vi "Pneumatics.vi"(7 "Solenoid Module":T2={"Unassigned"=enum."Solenoid 1", "Unassigned"=enum."Solenoid 2", "Arm In"=enum."Solenoid 3", "Arm Out"=enum."Solenoid 4", "MiniBot In"=enum."Solenoid 5", "MiniBot Out"=enum."Solenoid 6", "Unassigned"=enum."Solenoid 7", "Unassigned"=enum."Solenoid 8", "Switch and Relay Module"=enum."Solenoid Module 1"}, 8 "Mode":enum16{"Init", "Run", "End"}(ring), 10 "Inputs":T1) -> ()   [LabVIEW 2013]
doc: "This VI sets the pneumatics directly."
uses:
  Type Defs/Solenoid Module.ctl
  <vilib>/Rock Robotics/WPI/Solenoid/WPI_SolenoidChannel.ctl
  <vilib>/Rock Robotics/SystemInterfaces/Typedef/FPGA_TypedefSolenoidModule.ctl
  <vilib>/Rock Robotics/WPI/Solenoid/WPI_SolenoidValue.ctl
  <vilib>/Rock Robotics/WPI/Solenoid/WPI_SolenoidOpenDouble.vi
  <vilib>/Rock Robotics/WPI/Solenoid/WPI_SolenoidSetEnum.vi
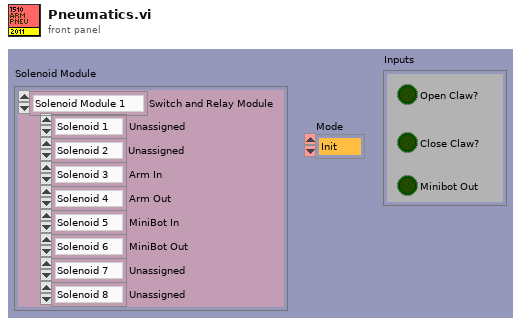
[diagram p1: front panel]
types:
  T1 = cluster{"Open Claw?":bool, "Close Claw?":bool, "Minibot Out":bool}
  T2 = typedef "Solenoid Module.ctl" = cluster{"Unassigned":T3, "Unassigned":T3, "Arm In":T3, "Arm Out":T3, "MiniBot In":T3, "MiniBot Out":T3, "Unassigned":T3, "Unassigned":T3, "Switch and Relay Module":T4}
  T3 = typedef "WPI_SolenoidChannel.ctl" = enum8{"Solenoid 1", "Solenoid 2", "Solenoid 3", "Solenoid 4", "Solenoid 5", "Solenoid 6", "Solenoid 7", "Solenoid 8", "Invalid"}
  T4 = typedef "FPGA_TypedefSolenoidModule.ctl" = enum16{"Solenoid Module 1", "Solenoid Module 2"}
  T5 = typedef "WPI_SolenoidValue.ctl" = enum16{"Off", "On", "Forward", "Reverse"}
  T6 = typedef "WPI_SolenoidDevRef.ctl" = cluster{"DevStatus":errorcluster, "Solenoid Module":T4, "Forward Solenoid Channel":T3, "Reverse Solenoid Channel":T3}
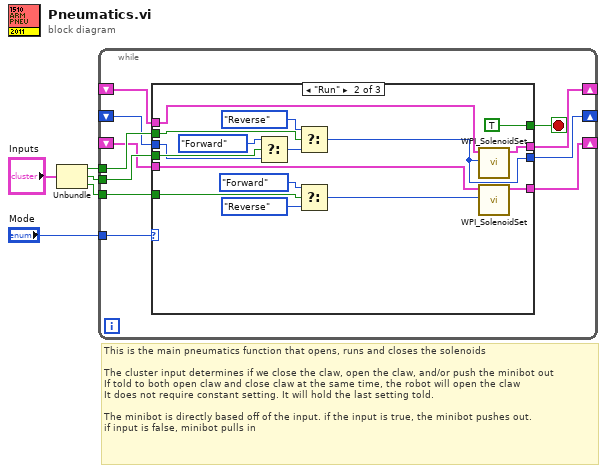
[diagram p0: block diagram]
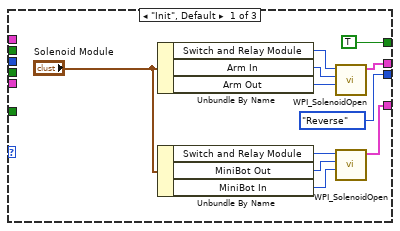
[diagram p2: hidden frame]
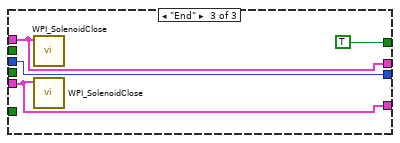
[diagram p3: hidden frame]
diagram:
  # "This is the main pneumatics function that opens, runs and closes the solenoids\n\nThe cluster input determines if we close the claw, open the claw, and/or push the minibot out\nIf told to both open claw and close claw at the same time, the robot will open the claw\nIt does not require constant setting. It will hold the last setting told.\n\nThe minibot is directly based off of the input. if the input is true, the minibot pushes out. \nif input is false, minibot pulls in"
  n1 = Unbundle("Inputs") -> ("Open Claw?"=w3:bool, "Close Claw?"=w2:bool, "Minibot Out"=w1:bool)
  n2 = while {
    tunnel: "Mode" -> [w16]
    shift-right: [w15] -> _
    shift-left: _ -> [w14]
    tunnel: w2 -> [w12]
    tunnel: w3 -> [w11]
    shift-right: [w8] -> _
    shift-left: _ -> [w10]
    tunnel: w1 -> [w9]
    shift-right: [w7] -> _
    shift-left: _ -> [w6]
    stop <- w13 stop-if-true
    n3 = case shown="\"Run\"" w16 {
      tunnel: [w27 w42 w47] -> w15
      tunnel: w14 -> [_ w43 w47]
      tunnel: [TRUE TRUE TRUE] -> w13
      tunnel: w12 -> [_ w40 _]
      tunnel: w11 -> [_ w38 _]
      tunnel: w10 -> [_ w35 w45]
      tunnel: w9 -> [_ w30 _]
      tunnel: [WPI_SolenoidValue."Reverse" ("t") w34 w45] -> w8
      tunnel: [w18 w28 w44] -> w7
      tunnel: w6 -> [_ w29 w44]
      frame "Init", Default {
        n4 = Unbundle By Name("Solenoid Module") -> ("Switch and Relay Module"=w23:T4, "Arm In"=w25:T3, "Arm Out"=w24:T3)
        n5 = Unbundle By Name("Solenoid Module") -> ("Switch and Relay Module"=w19:T4, "MiniBot Out"=w20:T3, "MiniBot In"=w21:T3)
        n6 = call-poly <vilib>:"WPI_SolenoidOpen.vi"("Reverse Solenoid Channel"=w24, "Forward Solenoid Channel"=w25, "Solenoid Module (Module 1)"=w23) -> ("SolenoidDevRef"=w27:T6)  [unwired: 1 in, 7 out]
        n7 = call-poly <vilib>:"WPI_SolenoidOpen.vi"("Reverse Solenoid Channel"=w21, "Forward Solenoid Channel"=w20, "Solenoid Module (Module 1)"=w19) -> ("SolenoidDevRef"=w18:T6)  [unwired: 1 in, 7 out]
      }
      frame "Run" {
        n8 = Select(t=WPI_SolenoidValue."Forward", s=w40, f=w35) -> (s? t:f=w39:T5)
        n9 = Select(t=WPI_SolenoidValue."Reverse", s=w38, f=w39) -> (s? t:f=w34:T5)
        n10 = Select(t=WPI_SolenoidValue."Forward" ("Value"), s=w30, f=WPI_SolenoidValue."Reverse" ("Value")) -> (s? t:f=w31:T5)
        n11 = call-poly <vilib>:"WPI_SolenoidSet.vi"("Value"=w34, "SolenoidDevRef"=w43) -> ("SolenoidDevRef"=w42:T6)  [unwired: 1 in, 8 out]
        n12 = call-poly <vilib>:"WPI_SolenoidSet.vi"("Value"=w31, "SolenoidDevRef"=w29) -> ("SolenoidDevRef"=w28:T6)  [unwired: 1 in, 8 out]
      }
      frame "End" {
        n13 = call <vilib>:"WPI_SolenoidClose.vi"("SolenoidDevRef"=w47) -> ()  [unwired: 1 in, 10 out]
        n14 = call <vilib>:"WPI_SolenoidClose.vi"("SolenoidDevRef"=w44) -> ()  [unwired: 1 in, 10 out]
      }
    }
  }
